vi "Base marwan_eleve.vi"() -> ()   [LabVIEW 2018]
uses:
  Global Humdidtiy 4.vi
  Global temperateurvi.vi
  Global  pressure.vi
  <vilib>/Instr/_visa.llb/VISA Configure Serial Port (Instr).vi
  <vilib>/express/express arith-compare/Formula/XNode/ExpressFormulaBlockNode.xnode
panel:
  in  "Path":path
  in  "OK Button":bool
  out "Chaîne 2":string
  out "Kelvin":dbl
  out "Fahrenheit":dbl
  in  "Pause":bool
  out "Moyen":dbl
  out "Moyen":dbl
  out "Moyen":dbl
  out "MAX":dbl
  out "MIN":dbl
  out "MIN":dbl
  out "MAX":dbl
  out "MIN":dbl
  out "MAX":dbl
  out "Waveform Humidity":dbl(graph)
  out "Waveform Pressure":dbl(graph)
  out "Waveform temperateur":dbl(graph)
  out "Humidity":dbl
  out "Pressure":dbl
  out "Temperateur":dbl
  out "Chaîne":string
  in  "stop":bool
  in  "Nom de ressource VISA":refnum<visa-resource-name>
  # "1. Brancher la carte Arduino sur un port USB\n2. Choisir le port COM de la carte dans la liste déroulante \"Nom de ressource VISA\"\n3. Lancer le programme"
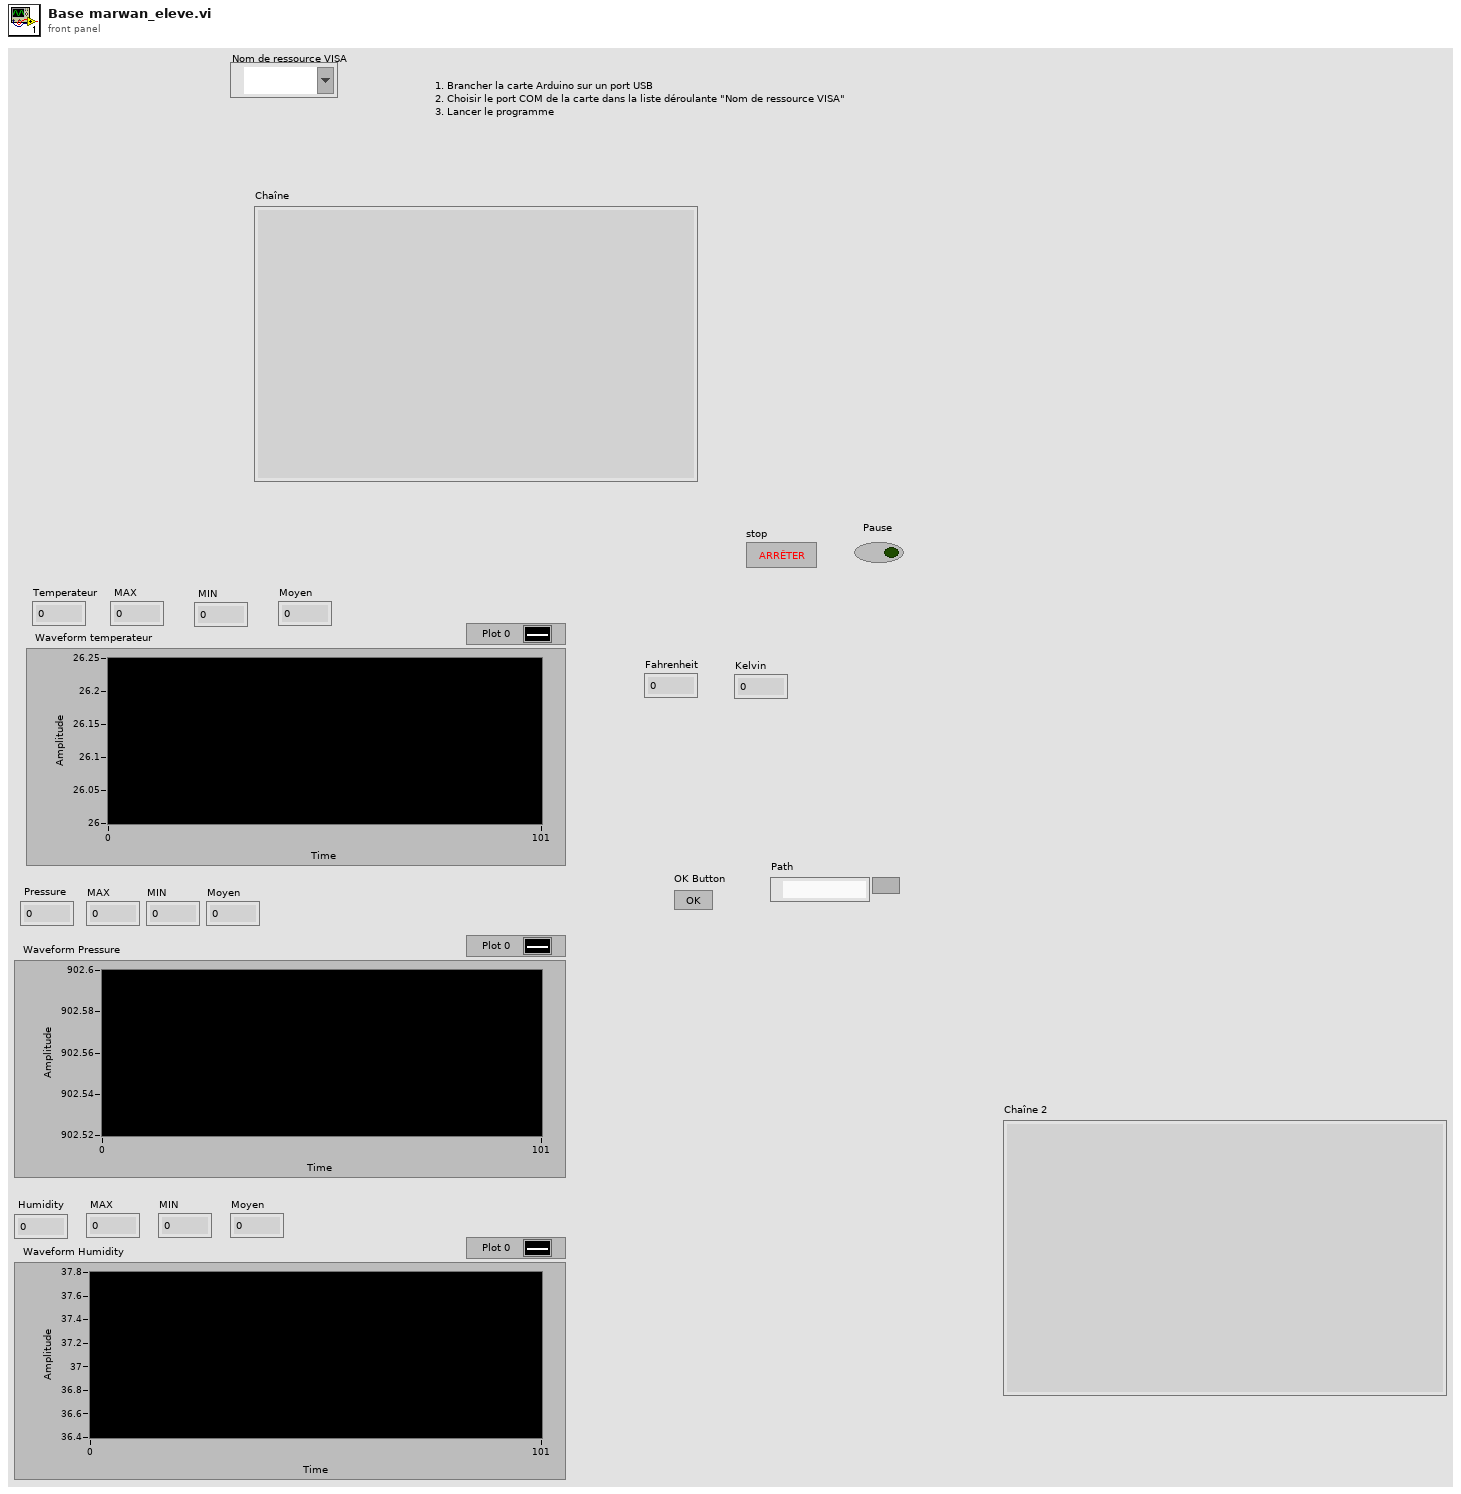
[diagram p1: front panel]
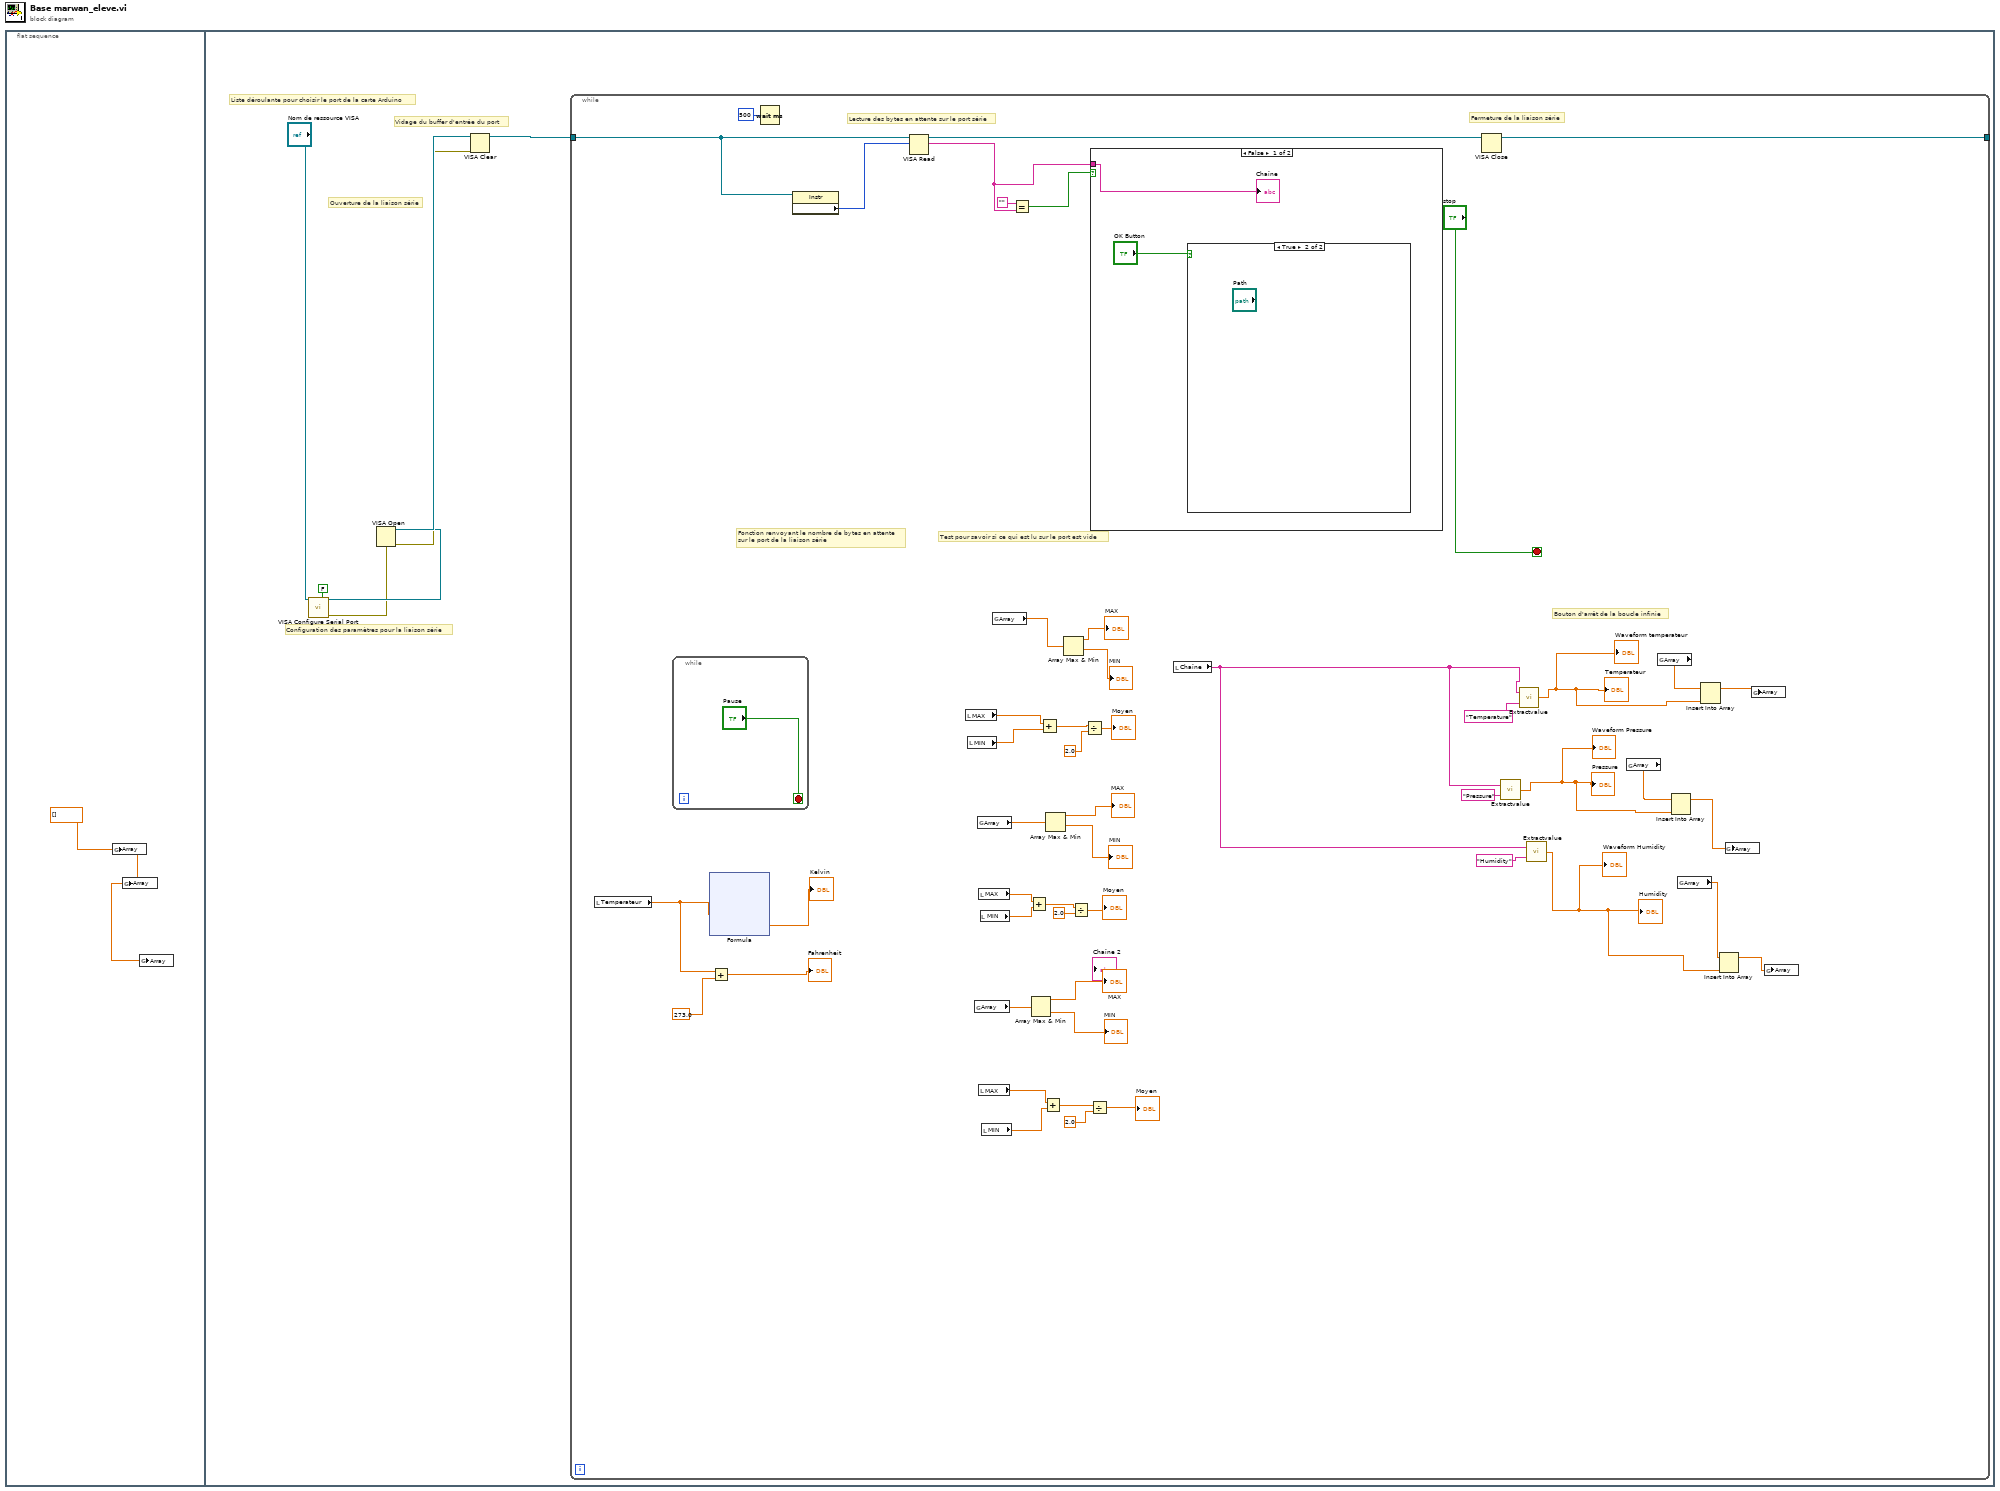
[diagram p0: block diagram]
diagram:
  n1 = flat-sequence {
    frame #0 {
      w1 = dbl[] []
      n2 = global write "Global  pressure.vi" "Array"(w1) -> ()
      n3 = global write "Global temperateurvi.vi" "Array"(w1) -> ()
      n4 = global write "Global Humdidtiy 4.vi" "Array"(w1) -> ()
    }
    frame #1 {
      # "Vidage du buffer d'entrée du port"
      # "Ouverture de la liaison série"
      # "Configuration des paramètres pour la liaison série"
      # "Liste déroulante pour choisir le port de la carte Arduino"
      # "Fermeture de la liaison série"
      n5 = call-poly "VISA Configure Serial Port"("VISA resource name"="Nom de ressource VISA", "Enable Termination\nChar (T)"=FALSE ("Enable Termination\nChar (T)")) -> ("VISA resource name out"=w6:refnum<visa-resource-name>, "error out"=w4:errorcluster)  [unwired: 12 in]
      n6 = VISA Open(error in (no error)=w4, VISA resource name=w6) -> (VISA resource name=w8:refnum<visa-resource-name>, error out=w3:errorcluster)  [unwired: 3 in]
      n7 = VISA Clear(VISA resource name=w8, error in (no error)=w3) -> (VISA resource name out=w7:refnum<visa-resource-name>)  [unwired: 1 out]
      n8 = while {
        tunnel: w7 -> [w57]
        tunnel: [w55] -> w2
        stop <- "stop" stop-if-true
        # "Lecture des bytes en attente sur le port série"
        # "Fonction renvoyant le nombre de bytes en attente\nsur le port de la liaison série"
        # "Test pour savoir si ce qui est lu sur le port est vide"
        # "Bouton d'arrêt de la boucle infinie"
        n9 = local read "Temperateur"() -> (w11:dbl)
        n10 = while {
          stop <- "Pause" stop-if-true
        }
        n11 = xnode "Formula"("X1"=w11) -> ("Result"=→"Kelvin":dbl)  [unwired: 1 in, 1 out]
        n12 = Add(x=w11, y=273.0) -> (x+y=→"Fahrenheit":dbl)
        n13 = Wait (ms)(milliseconds to wait=u32 500 ("attente (ms)")) -> ()  [unwired: 1 out]
        n14 = property class="Instr"(reference=w57) -> ("Serial Settings:Number of Bytes at Serial Port"=w56:u32)  [unwired: 1 in, 2 out]
        n15 = VISA Read(VISA resource name=w57, byte count=w56) -> (VISA resource name out=w55:refnum<visa-resource-name>, read buffer=w51:string)  [unwired: 1 in, 2 out]
        n16 = local read "MAX"() -> (w28:dbl)
        n17 = local read "MIN"() -> (w27:dbl)
        n18 = global read "Global Humdidtiy 4.vi" "Array"() -> (w31:dbl[])
        n19 = global read "Global  pressure.vi" "Array"() -> (w38:dbl[])
        n20 = local read "MAX"() -> (w23:dbl)
        n21 = local read "MAX"() -> (w18:dbl)
        n22 = local read "MIN"() -> (w22:dbl)
        n23 = local read "MIN"() -> (w17:dbl)
        n24 = global read "Global temperateurvi.vi" "Array"() -> (w43:dbl[])
        n25 = Equal?(x="", y=w51) -> (x = y?=w52:bool)
        n26 = Add(x=w23, y=w22) -> (x+y=w21:dbl)
        n27 = Array Max & Min(array=w31) -> (max value=→"MAX":dbl, min value=→"MIN":dbl)  [unwired: 2 out]
        n28 = Add(x=w28, y=w27) -> (x+y=w26:dbl)
        n29 = Add(x=w18, y=w17) -> (x+y=w16:dbl)
        n30 = Array Max & Min(array=w38) -> (max value=→"MAX":dbl, min value=→"MIN":dbl)  [unwired: 2 out]
        n31 = Array Max & Min(array=w43) -> (max value=→"MAX":dbl, min value=→"MIN":dbl)  [unwired: 2 out]
        n32 = Divide(x=w21, y=2.0) -> (x/y=→"Moyen":dbl)
        n33 = Divide(x=w26, y=2.0) -> (x/y=→"Moyen":dbl)
        n34 = Divide(x=w16, y=2.0) -> (x/y=→"Moyen":dbl)
        n35 = case shown="False" w52 {
          tunnel: w51 -> [w69 _]
          frame False {
            n36 = case shown="True" "OK Button" {
              frame False {
              }
              frame True {
              }
            }
            "Chaîne" <- w69
          }
          frame True {
          }
        }
        n37 = local read "Chaîne"() -> (w47:string)
        n38 = call "Extractvalue.vi"("Mesure"="Pressure", "Chaîne"=w47) -> ("Value"=w40:dbl)
        "Pressure" <- w40
        "Waveform Pressure" <- w40
        n39 = call "Extractvalue.vi"("Mesure"="Temperature", "Chaîne"=w47) -> ("Value"=w45:dbl)
        "Temperateur" <- w45
        "Waveform temperateur" <- w45
        n40 = call "Extractvalue.vi"("Mesure"="Humidity", "Chaîne"=w47) -> ("Value"=w34:dbl)
        "Humidity" <- w34
        "Waveform Humidity" <- w34
        n41 = global read "Global  pressure.vi" "Array"() -> (w35:dbl[])
        n42 = global read "Global temperateurvi.vi" "Array"() -> (w46:dbl[])
        n43 = Insert Into Array(array=w35, new element=w40) -> (w39:dbl[])  [unwired: 1 in]
        n44 = global read "Global Humdidtiy 4.vi" "Array"() -> (w33:dbl[])
        n45 = Insert Into Array(array=w46, new element=w45) -> (w44:dbl[])  [unwired: 1 in]
        n46 = Insert Into Array(array=w33, new element=w34) -> (w32:dbl[])  [unwired: 1 in]
        n47 = global write "Global  pressure.vi" "Array"(w39) -> ()
        n48 = global write "Global temperateurvi.vi" "Array"(w44) -> ()
        n49 = global write "Global Humdidtiy 4.vi" "Array"(w32) -> ()
      }
      n50 = VISA Close(VISA resource name=w2) -> ()  [unwired: 1 in, 1 out]
    }
  }
